vi "day1-2.vi"() -> ()   [LabVIEW 2021]
uses:
  <vilib>/Utility/file.llb/Read Delimited Spreadsheet (string).vi
panel:
  in  "Example":string="1000\n2000\n3000\n\n4000\n\n5000\n6000\n\n7000\n8000\n9000\n\n10000"
  in  "Example":bool
  out "Answer":i32=211447
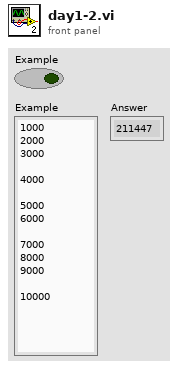
[diagram p1: front panel]
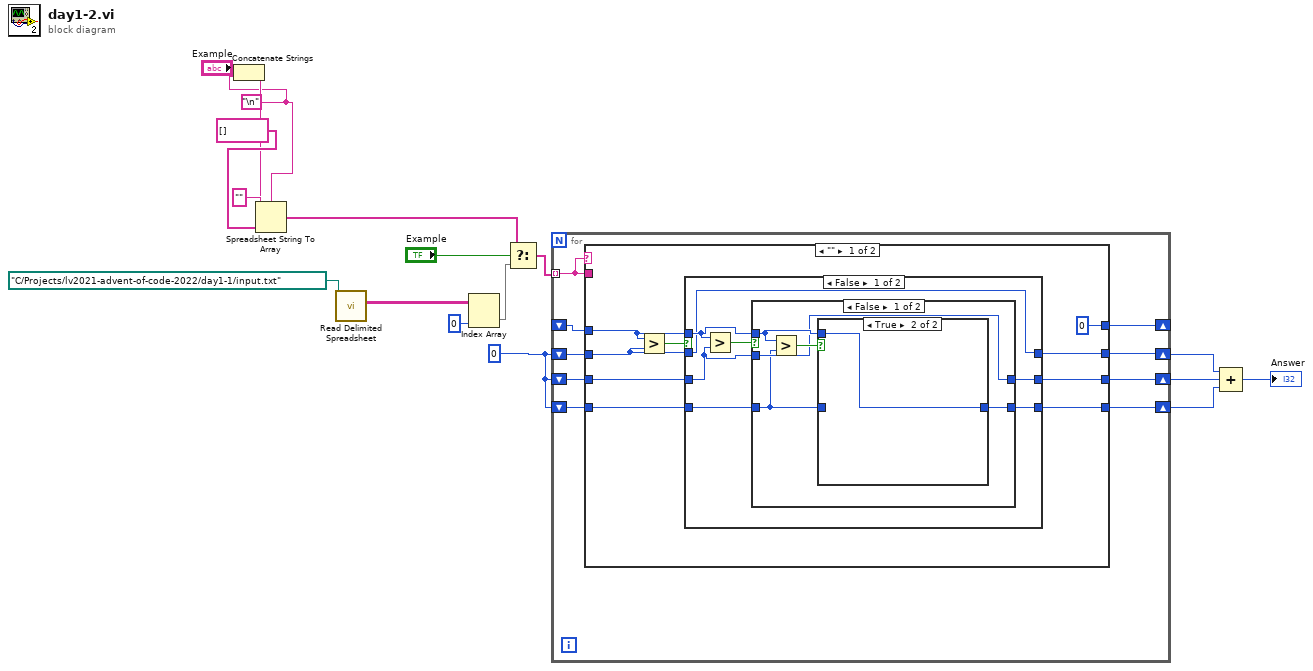
[diagram p0: block diagram]
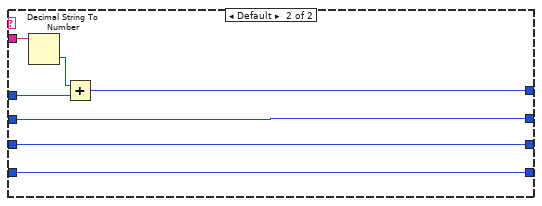
[diagram p5: hidden frame]
diagram:
  w7 = 0
  w1 = "\n"
  n1 = Concatenate Strings("Example", w1) -> (w2:string)
  n2 = Spreadsheet String To Array(delimiter (Tab)=w1, format string="", spreadsheet string=w2, array type (2D Dbl)=string[] [] ("t")) -> (array=w9:string[])
  n3 = call-poly <vilib>:"Read Delimited Spreadsheet.vi"("file path (dialog if empty)"=path "C:/Projects/lv2021-advent-of-code-2022/day1-1/input.txt") -> ("all rows"=w16:string[][])  [unwired: 9 in, 5 out]
  n4 = Index Array(array=w16, index (col)=0 ("disabled index (col)")) -> (element=w14:string[])  [unwired: 1 in]
  n5 = Select(t=w9, s="Example", f=w14) -> (s? t:f=w13:string[])
  n6 = for {
    tunnel: w13 -> [w24] mode=indexing
    shift-right: [w26] -> _
    shift-left: _ -> [w25]
    shift-right: [w23] -> w5
    shift-left: w7 -> [w22]
    shift-right: [w19] -> w6
    shift-left: w7 -> [w21]
    shift-right: [w18] -> w4
    shift-left: w7 -> [w20]
    n7 = case shown="\"\"" w24 {
      tunnel: [0 w61] -> w26
      tunnel: w25 -> [w32 w60]
      tunnel: w24 -> [_ w58]
      tunnel: [w34 w57] -> w23
      tunnel: w22 -> [w31 w57]
      tunnel: w21 -> [w30 w56]
      tunnel: w20 -> [w29 w55]
      tunnel: [w28 w56] -> w19
      tunnel: [w27 w55] -> w18
      frame "" {
        n8 = Greater?(x=w32, y=w31) -> (0:w33:bool)
        n9 = case shown="False" w33 {
          tunnel: [w38 w54] -> w34
          tunnel: w32 -> [w39 w54]
          tunnel: w31 -> [w38 w53]
          tunnel: w30 -> [w40 w52]
          tunnel: w29 -> [w41 _]
          tunnel: [w37 w53] -> w28
          tunnel: [w36 w52] -> w27
          frame False {
            n10 = Greater?(x=w39, y=w40) -> (0:w42:bool)
            n11 = case shown="False" w42 {
              tunnel: w41 -> [w43 _]
              tunnel: w40 -> [w45 w50]
              tunnel: w39 -> [w46 w51]
              tunnel: [w45 w51] -> w37
              tunnel: [w44 w50] -> w36
              frame False {
                n12 = Greater?(x=w46, y=w43) -> (0:w47:bool)
                n13 = case shown="True" w47 {
                  tunnel: w46 -> [_ w49]
                  tunnel: [w48 w49] -> w44
                  tunnel: w43 -> [w48 _]
                  frame False {
                  }
                  frame True {
                  }
                }
              }
              frame True {
              }
            }
          }
          frame True {
          }
        }
      }
      frame Default {
        n14 = Decimal String To Number(string=w58) -> (number=w59:i32)  [unwired: 2 in, 1 out]
        n15 = Add(x=w59, y=w60) -> (x+y=w61:i32)
      }
    }
  }
  n16 = Compound Arithmetic op=ADD(w5, w6, w4) -> (→"Answer":i32)
